vi "Create Tree Shortcut Menu.vi"(10 "Selection":T1=enum."» Public API VIs", 11 "Menu in":refnum<k9>) -> (0 "error out":errorcluster)   [LabVIEW 2020, in "Panther Dashboard.lvlib"]
uses:
  Panther Dashboard.lvlib
  Class/LabVIEWItem/Item Type--enum.ctl
  Panther Dashboard--global.vi
  Class/LabVIEWItem/LabVIEWItem.lvclass
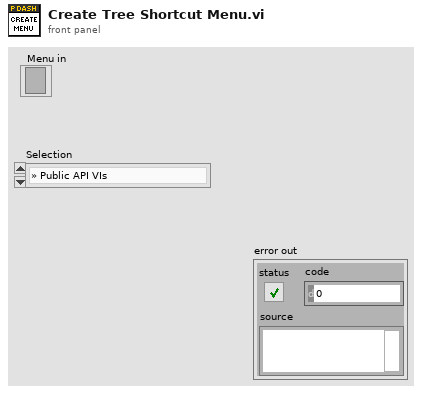
[diagram p1: front panel]
types:
  T1 = typedef "Panther Dashboard.lvlib/LabVIEWItem.lvclass/Item Type--enum.ctl" = enum16{"Requests", "Broadcasts", "Request and Wait for Reply", "Round Trip", "» Public API VIs", "» Constant VIs", "» Error VIs", "Module", "Project", "No Drag Selection"}
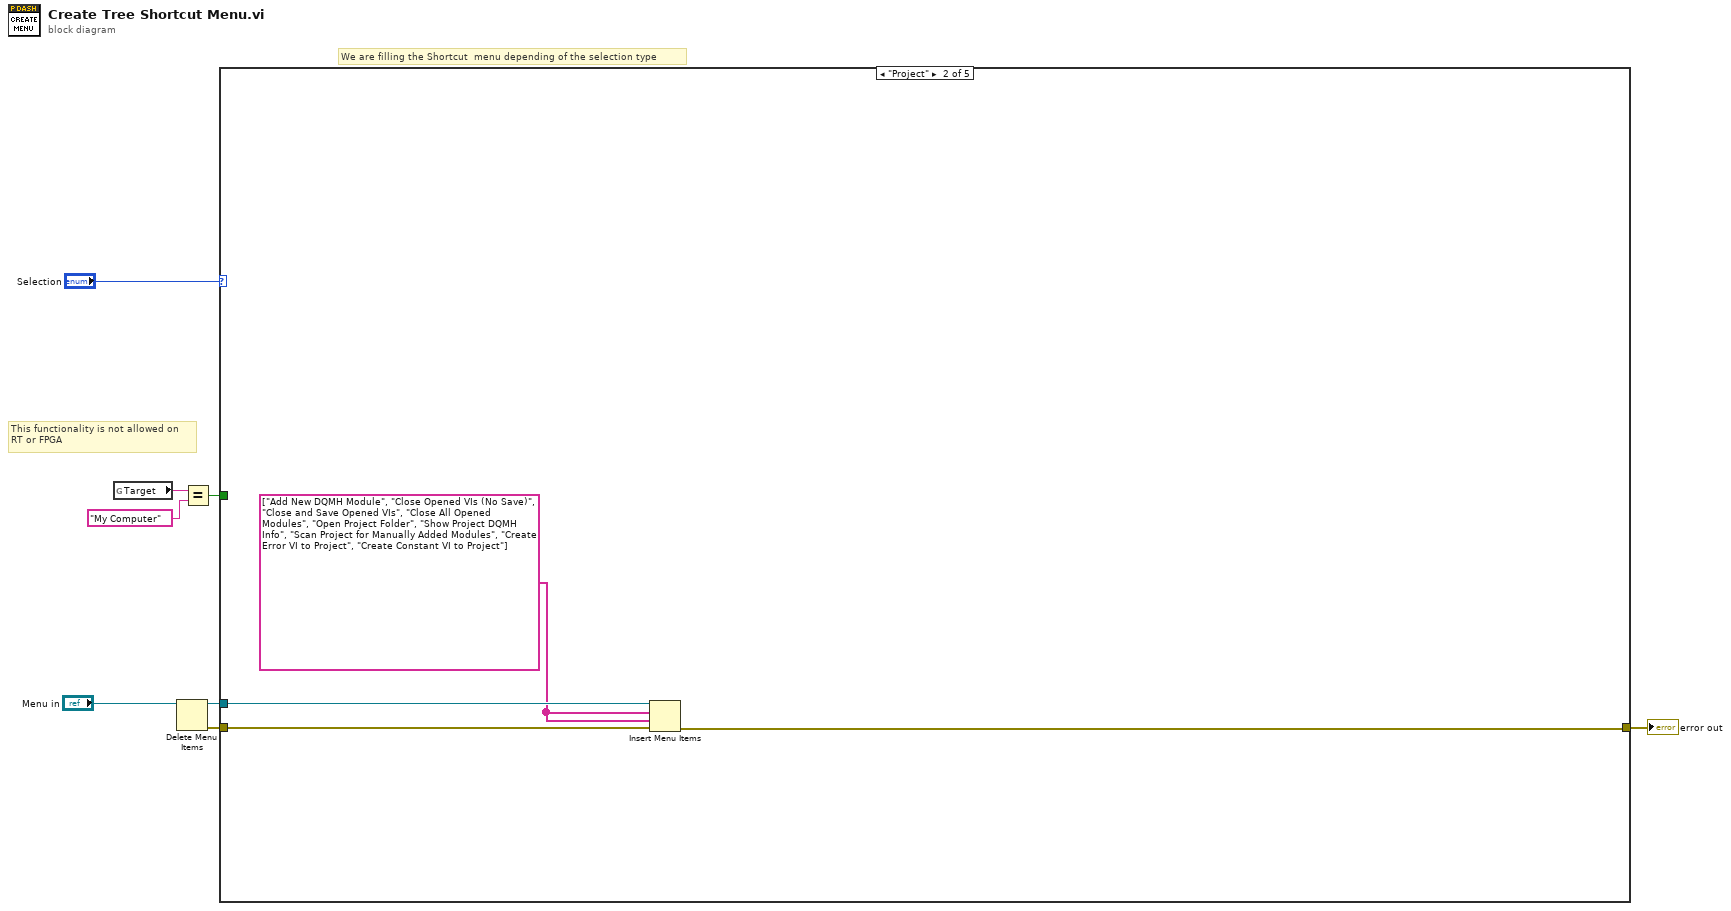
[diagram p0: block diagram]
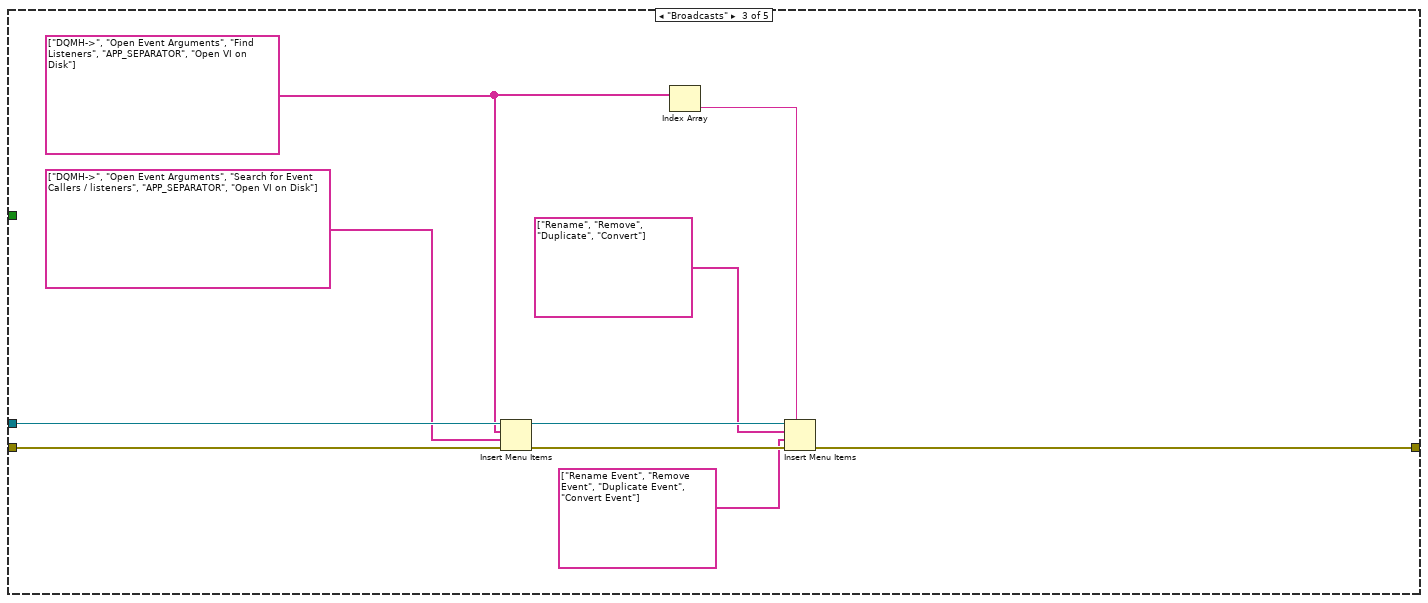
[diagram p3: hidden frame]
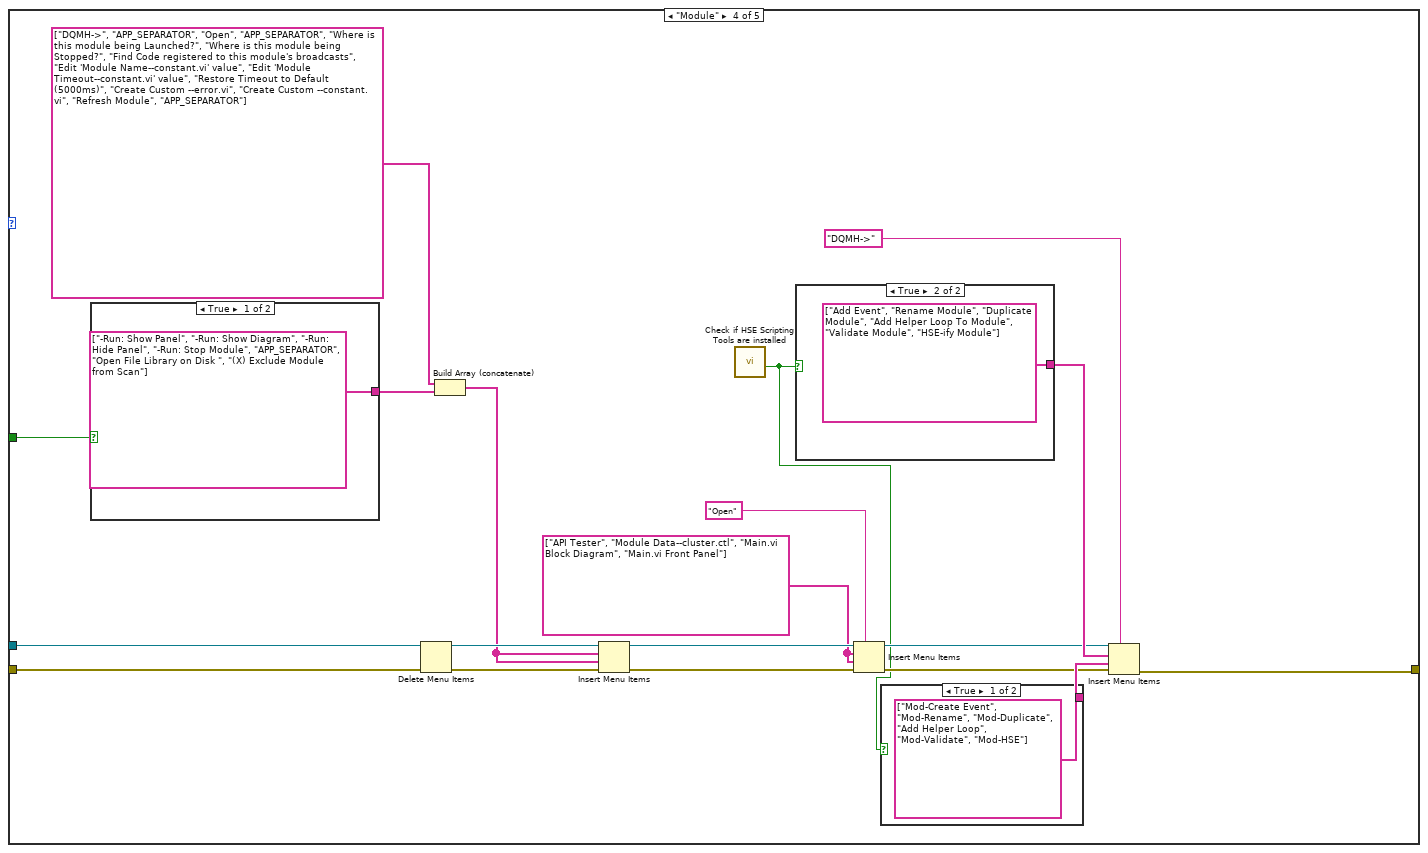
[diagram p4: hidden frame]
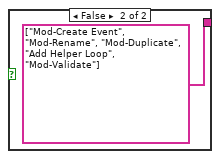
[diagram p5: hidden frame]
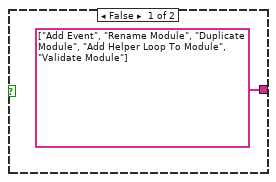
[diagram p6: hidden frame]
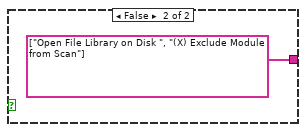
[diagram p7: hidden frame]
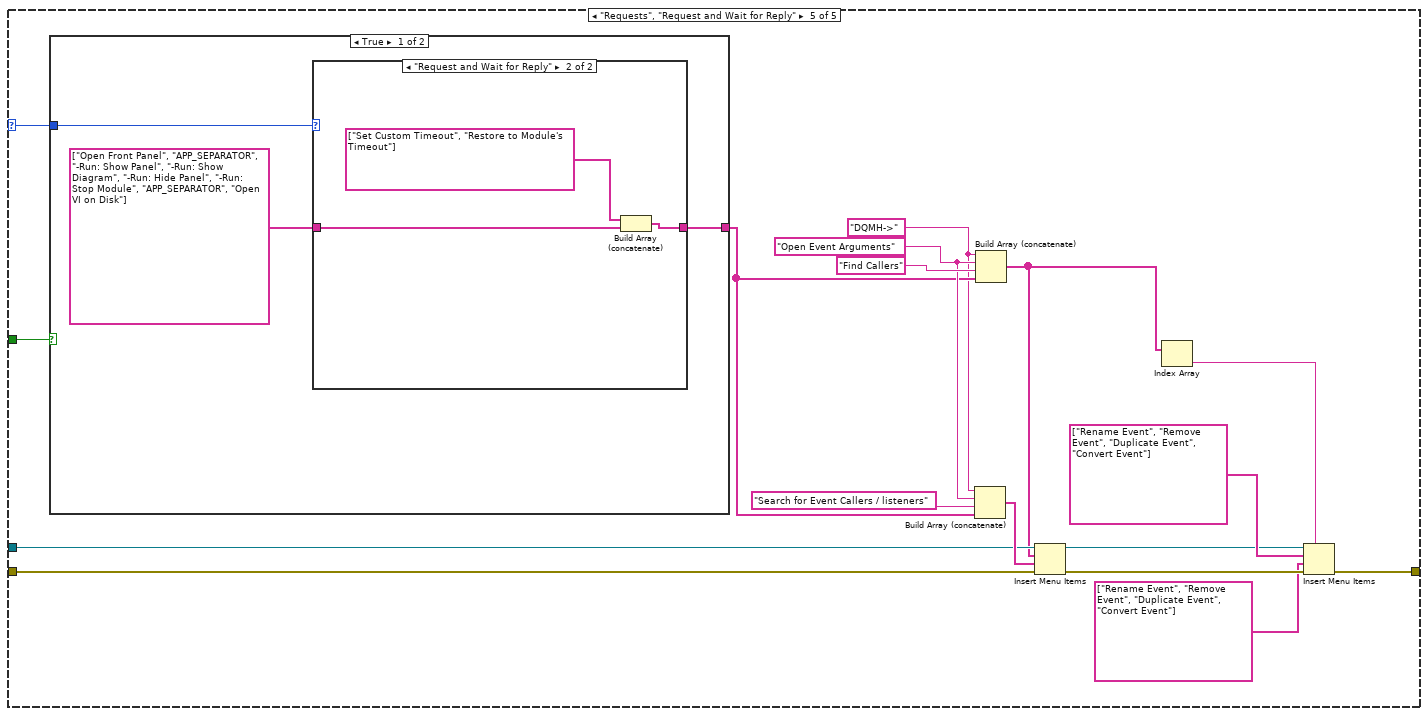
[diagram p8: hidden frame]
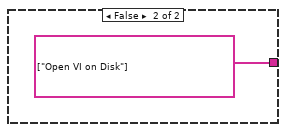
[diagram p10: hidden frame]
diagram:
  # "This functionality is not allowed on\nRT or FPGA"
  # "We are filling the Shortcut  menu depending of the selection type"
  n1 = global read "Panther Dashboard--global.vi" "Target"() -> (w4:string)
  n2 = Delete Menu Items(9:"Menu in") -> (0:w7:errorcluster, 3:w5:refnum<k9>)  [unwired: 3 in]
  n3 = Equal?(x=w4, y="My Computer") -> (x = y?=w2:bool)
  n4 = case shown="\"Project\"" "Selection" {
    selector: "Selection" -> [_ _ _ _ w55]
    tunnel: [w9 w13 w21 w39 w63] -> w8
    tunnel: w7 -> [w9 w12 w22 w41 w65]
    tunnel: w5 -> [_ w11 w20 w35 w59]
    tunnel: w2 -> [_ _ _ w34 w58]
    frame Default {
    }
    frame "Project" {
      w10 = string[] ["Add New DQMH Module", "Close Opened VIs (No Save)", "Close and Save Opened VIs", "Close All Opened Modules", "Open Project Folder", "Show Project DQMH Info", "Scan Project for Manually Added Modules", "Create Error VI to Project", "Create Constant VI to Project"] ("item names")
      n5 = Insert Menu Items(6:w12, 7:w10, 8:w10, 9:w11) -> (0:w13:errorcluster)  [unwired: 2 in, 2 out]
    }
    frame "Broadcasts" {
      w17 = string[] ["DQMH->", "Open Event Arguments", "Find Listeners", "APP_SEPARATOR", "Open VI on Disk"]
      n6 = Insert Menu Items(6:w22, 7:string[] ["DQMH->", "Open Event Arguments", "Search for Event Callers / listeners", "APP_SEPARATOR", "Open VI on Disk"], 8:w17, 9:w20) -> (0:w23:errorcluster, 3:w18:refnum<k9>)  [unwired: 2 in, 1 out]
      n7 = Index Array(array=w17) -> (element=w16:string)  [unwired: 1 in]
      n8 = Insert Menu Items(5:w16, 6:w23, 7:string[] ["Rename Event", "Remove Event", "Duplicate Event", "Convert Event"] ("item names"), 8:string[] ["Rename", "Remove", "Duplicate", "Convert"] ("item names"), 9:w18) -> (0:w21:errorcluster)  [unwired: 1 in, 2 out]
    }
    frame "Module" {
      w27 = string[] ["API Tester", "Module Data--cluster.ctl", "Main.vi Block Diagram", "Main.vi Front Panel"] ("item names")
      n9 = case shown="True" w34 {
        tunnel: [string[] ["-Run: Show Panel", "-Run: Show Diagram", "-Run: Hide Panel", "-Run: Stop Module", "APP_SEPARATOR", "Open File Library on Disk ", "(X) Exclude Module from Scan"] ("item names") string[] ["Open File Library on Disk ", "(X) Exclude Module from Scan"] ("item names")] -> w37
        frame True {
        }
        frame False {
        }
      }
      n10 = Delete Menu Items(6:w41, 9:w35) -> (0:w42:errorcluster, 3:w38:refnum<k9>)  [unwired: 2 in]
      n11 = Build Array (concatenate)(string[] ["DQMH->", "APP_SEPARATOR", "Open", "APP_SEPARATOR", "Where is this module being Launched?", "Where is this module being Stopped?", "Find Code registered to this module's broadcasts", "Edit 'Module Name--constant.vi' value", "Edit 'Module Timeout--constant.vi' value", "Restore Timeout to Default (5000ms)", "Create Custom --error.vi", "Create Custom --constant.vi", "Refresh Module", "APP_SEPARATOR"] ("item names"), w37) -> (w36:string[])
      n12 = Insert Menu Items(6:w42, 7:w36, 8:w36, 9:w38) -> (0:w40:errorcluster, 3:w29:refnum<k9>)  [unwired: 2 in, 1 out]
      n13 = call "Check if HSE Scripting Tools are installed.vi"() -> ("HSE Scripting tools Installed?"=w24:bool)  [unwired: 10 in, 1 out]
      n14 = case shown="True" w24 {
        tunnel: [string[] ["Add Event", "Rename Module", "Duplicate Module", "Add Helper Loop To Module", "Validate Module"] ("item names") string[] ["Add Event", "Rename Module", "Duplicate Module", "Add Helper Loop To Module", "Validate Module", "HSE-ify Module"] ("item names")] -> w32
        frame False {
        }
        frame True {
        }
      }
      n15 = Insert Menu Items(5:"Open" ("menu tag"), 6:w40, 7:w27, 8:w27, 9:w29) -> (0:w30:errorcluster, 3:w28:refnum<k9>)  [unwired: 1 in, 1 out]
      n16 = case shown="True" w24 {
        tunnel: [string[] ["Mod-Create Event", "Mod-Rename", "Mod-Duplicate", "Add Helper Loop", "Mod-Validate", "Mod-HSE"] ("item names") string[] ["Mod-Create Event", "Mod-Rename", "Mod-Duplicate", "Add Helper Loop", "Mod-Validate"] ("item names")] -> w31
        frame True {
        }
        frame False {
        }
      }
      n17 = Insert Menu Items(5:"DQMH->" ("menu tag"), 6:w30, 7:w31, 8:w32, 9:w28) -> (0:w39:errorcluster)  [unwired: 1 in, 2 out]
    }
    frame "Requests", "Request and Wait for Reply" {
      w49 = "DQMH->" ("element")
      w57 = "Open Event Arguments"
      n18 = case shown="True" w58 {
        tunnel: [w67 string[] ["Open VI on Disk"] ("item names")] -> w56
        tunnel: w55 -> [w66 _]
        frame True {
          n19 = case shown="\"Request and Wait for Reply\"" w66 {
            tunnel: string[] ["Open Front Panel", "APP_SEPARATOR", "-Run: Show Panel", "-Run: Show Diagram", "-Run: Hide Panel", "-Run: Stop Module", "APP_SEPARATOR", "Open VI on Disk"] ("item names") -> [w69 w70]
            tunnel: [w69 w71] -> w67
            frame Default {
            }
            frame "Request and Wait for Reply" {
              n20 = Build Array (concatenate)(string[] ["Set Custom Timeout", "Restore to Module's Timeout"], w70) -> (w71:string[])
            }
          }
        }
        frame False {
        }
      }
      n21 = Build Array (concatenate)(w49, w57, "Search for Event Callers / listeners", w56) -> (w61:string[])
      n22 = Build Array (concatenate)(w49, w57, "Find Callers", w56) -> (w50:string[])
      n23 = Insert Menu Items(6:w65, 7:w61, 8:w50, 9:w59) -> (0:w64:errorcluster, 3:w51:refnum<k9>)  [unwired: 2 in, 1 out]
      n24 = Index Array(array=w50) -> (element=w54:string)  [unwired: 1 in]
      n25 = Insert Menu Items(5:w54, 6:w64, 7:string[] ["Rename Event", "Remove Event", "Duplicate Event", "Convert Event"] ("item names"), 8:string[] ["Rename Event", "Remove Event", "Duplicate Event", "Convert Event"] ("item names"), 9:w51) -> (0:w63:errorcluster)  [unwired: 1 in, 2 out]
    }
  }
  "error out" <- w8
